vi "Call Library.vi"   [LabVIEW 2023]
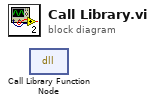
[diagram p0: block diagram]
diagram:
  n1 = dll-call lib="gfitsio.dll" fn="Call Library Function Node"() -> ()  [unwired: 4 in, 2 out]
